vi "Format Log.vi"(0 "error handler in":refnum<class "TLB` Error Handler.lvclass">, 11 "error in":errorcluster) -> (4 "error handler out":refnum<class "TLB` Error Handler.lvclass">, 6 "source text":string, 15 "error out":errorcluster)   [LabVIEW 2018, in "Springboard TLB`.lvlib" / "TLB` Error Handler.lvclass"]
uses:
  TLB` Error Handler.lvclass
  TLB` Error Handler.lvclass/TLB` Error Handler.ctl
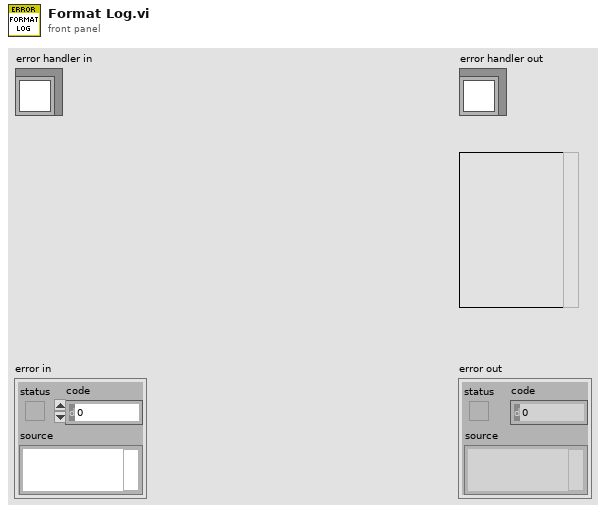
[diagram p1: front panel]
types:
  T1 = typedef "Springboard TLB`.lvlib/TLB` Error Handler.lvclass/Log Action.ctl" = enum16{"Default", "Override", "Appended to Beginning", "Append to End"}
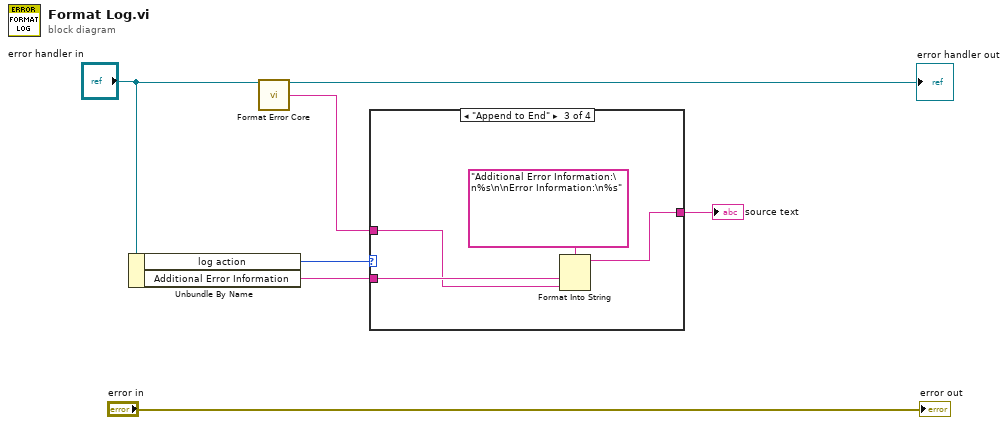
[diagram p0: block diagram]
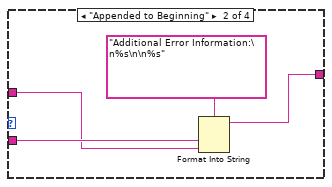
[diagram p3: hidden frame]
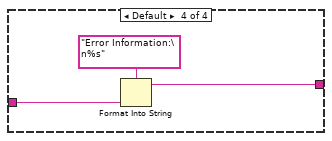
[diagram p4: hidden frame]
diagram:
  n1 = Unbundle By Name("error handler in") -> ("log action"=w3:T1, "Additional Error Information"=w1:string)
  n2 = call "Format Error Core.vi"("error handler in"="error handler in") -> ("error handler out"=→"error handler out":refnum<class "TLB` Error Handler.lvclass">, "source text"=w5:string)  [unwired: 13 in]
  n3 = case shown="\"Append to End\"" w3 {
    tunnel: w5 -> [_ w10 w14 w19]
    tunnel: [w8 w9 w13 w18] -> w2
    tunnel: w1 -> [w8 w12 w16 _]
    frame "Override" {
    }
    frame "Appended to Beginning" {
      n4 = Format Into String(format string="Additional Error Information:\n%s\n\n%s", w12, w10) -> (resulting string=w9:string)  [unwired: 2 in, 1 out]
    }
    frame "Append to End" {
      n5 = Format Into String(format string="Additional Error Information:\n%s\n\nError Information:\n%s", w16, w14) -> (resulting string=w13:string)  [unwired: 2 in, 1 out]
    }
    frame Default {
      n6 = Format Into String(format string="Error Information:\n%s", w19) -> (resulting string=w18:string)  [unwired: 2 in, 1 out]
    }
  }
  "source text" <- w2
  "error out" <- "error in"
